vi "Motor with Encoder - Bang Bang.vi"() -> ()   [LabVIEW 2016]
doc: "This example shows how to move a motor connected to an encoder and a wheel, and then read information about the system from an encoder.\n\nThis is an example of how to use feedback (from the encoder) to create an open loop system. If some control method was used, for example using PID, a closed loop system could be created.\n\nThis example expects a USB cable connected from your development PC to the Type B USB Jack (next to the power input) on the roboRIO.\n\nThis example requires the Driver Station to be running with Teleoperated Enabled."
uses:
  <vilib>/Rock Robotics/SystemInterfaces/DIO/FPGA_DIOChannel.ctl
  <vilib>/Rock Robotics/WPI/Encoder/WPI_EncoderType.ctl
  <vilib>/Rock Robotics/SystemInterfaces/DIO/FPGA_DIOPWMChannel.ctl
  <vilib>/Rock Robotics/WPI/Counter/WPI_CounterDigitalInputToDigitalSource.vi
  <vilib>/Rock Robotics/WPI/MotorControl/WPI_MotorControlOpen SPARK.vi
  <vilib>/gmath/NI_Gmath.lvlib
panel:
  in  "Encoder Before Gearbox":bool
  in  "Update RPM":bool
  in  "Error Multiplication Value":dbl
  in  "Lower Limit":dbl=-50.0 format="%#_13g"
  in  "Upper Limit":dbl=50.0 format="%#_13g"
  out "Error":dbl(graph)=-19.827905182603445
  out "Error":dbl=-19.827905182603445
  out "DS Original":dbl=0.6428571428571428
  in  "Neg Drive Signal":dbl=0.6
  in  "Pos Drive Signal":dbl=1.0
  in  "Target RPM":dbl=3300.0
  in  "MS to Wait":u32=10
  out "Loop Time (s)":dbl=0.010378 format="%_6f"
  out "RPM":dbl=3319.8279051826034
  out "XY Graph":cluster{dbl[], dbl[]}[](graph)
  out "Waveform Chart":dbl(graph)=3319.8279051826034
  in  "Motor PWM Channel":T1=enum."PWM 9"
  in  "Number Samples to Average":u8=1 min=1 max=128
  in  "Invert Direction":bool=TRUE
  in  "Decoding Type":T2=enum."2x"
  in  "DistancePerCount (deg)":dbl=0.351563
  in  "Encoder B Channel":T3=enum."DIO 1"
  in  "Encoder A Channel":T3
  in  "Minimum Rate":dbl=20.0
  in  "Stop":bool
  out "Encoder Alarm Status":string="Encoder Moving"
  out "Encoder Direction":string="Forward"
  # "These can be set while running."
  # "Output information."
  # "Set these inputs before running."
  # "This example requires the Driver Station to be running with Teleoperated Enabled."
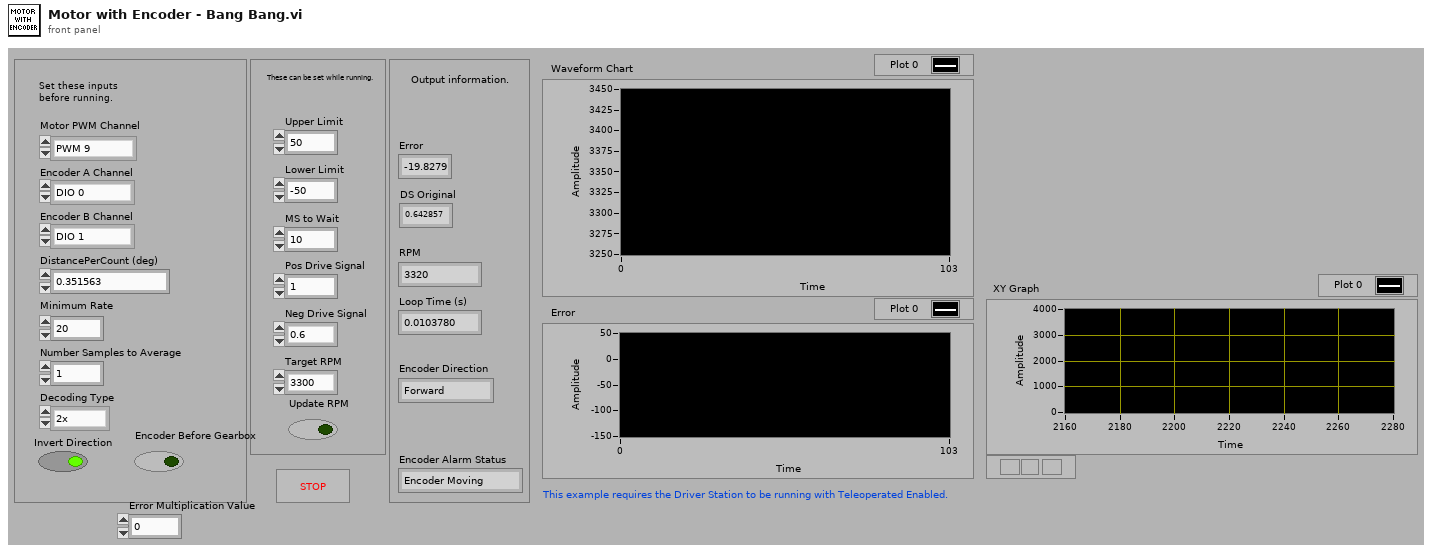
[diagram p1: front panel]
types:
  T1 = typedef "FPGA_DIOPWMChannel.ctl" = enum8{"PWM 0", "PWM 1", "PWM 2", "PWM 3", "PWM 4", "PWM 5", "PWM 6", "PWM 7", "PWM 8", "PWM 9", "PWM MXP 0", "PWM MXP 1", "PWM MXP 2", "PWM MXP 3", "PWM MXP 4", "PWM MXP 5", "PWM MXP 6", "PWM MXP 7", "PWM MXP 8", "PWM MXP 9", "Invalid"}
  T2 = typedef "WPI_EncoderType.ctl" = enum16{"1x", "2x", "4x"}
  T3 = typedef "FPGA_DIOChannel.ctl" = enum8{"DIO 0", "DIO 1", "DIO 2", "DIO 3", "DIO 4", "DIO 5", "DIO 6", "DIO 7", "DIO 8", "DIO 9", "DIO MXP 0", "DIO MXP 1", "DIO MXP 2", "DIO MXP 3", "DIO MXP 4", "DIO MXP 5", "DIO MXP 6", "DIO MXP 7", "DIO MXP 8", "DIO MXP 9", "DIO MXP 10", "DIO MXP 11", "DIO MXP 12", "DIO MXP 13", "DIO MXP 14", "DIO MXP 15", "SPI Port CS1", "SPI Port CS2", "SPI Port CS3", "SPI Port MISO", "SPI Port MOSI", "Invalid"}
  T4 = typedef "WPI_MotorControlDeviceRef.ctl" = cluster{"DeviceStatus":errorcluster, "Type":T5, "PWM":cluster{"PWM Channel":T1, "DeadBand":T6}, "CAN":cluster{"Device Number":u8, "SetOutput VI Ref":variant, "GetOutput VI Ref":variant, "Enable VI Ref":variant, "Disable VI Ref":variant, "Data":variant}, "Invert":bool}
  T5 = typedef "WPI_MotorControlType.ctl" = enum16{"PWM", "CAN"}
  T6 = typedef "WPI_PWMDeadband.ctl" = cluster{"Name":string, "maxPositivePwm":i32, "minPositivePwm":i32, "centerPwm":i32, "maxNegativePwm":i32, "minNegativePwm":i32, "angularRange":u16}
  T7 = typedef "WPI_DigitalInputDevRef.ctl" = cluster{"DevStatus":errorcluster, "DIO Channel":T3}
  T8 = typedef "FPGA_CounterEncoderSourceConvertionLVSourceType.ctl" = cluster{"DevStatus":errorcluster, "AnalogTriggerMode?":bool, "DigitalMode":cluster{"DIO Channel":T9}, "AnalogTriggerMode":cluster{"AnalogTriggerIndex":T10, "OutputType":T11}}
  T9 = typedef "FPGA_DIODigitalSourceChannel.ctl" = enum8{"DIO 0", "DIO 1", "DIO 2", "DIO 3", "DIO 4", "DIO 5", "DIO 6", "DIO 7", "DIO 8", "DIO 9", "DIO MXP 0", "DIO MXP 1", "DIO MXP 2", "DIO MXP 3", "DIO MXP 4", "DIO MXP 5", "DIO MXP 6", "DIO MXP 7", "DIO MXP 8", "DIO MXP 9", "DIO MXP 10", "DIO MXP 11", "DIO MXP 12", "DIO MXP 13", "DIO MXP 14", "DIO MXP 15", "Disabled"}
  T10 = typedef "FPGA_AnalogTriggerIndex.ctl" = enum8{"Trig 0", "Trig 1", "Trig 2", "Trig 3", "Trig 4", "Trig 5", "Trig 6", "Trig 7", "Invalid"}
  T11 = typedef "FPGA_AnalogTriggerOutType.ctl" = enum16{"InWindow", "TriggerState", "Rising", "Falling"}
  T12 = typedef "WPI_EncoderDevRef.ctl" = cluster{"DevStatus":errorcluster, "EncoderIndex":T13, "CounterIndex":T14, "DistancePerCount":dbl, "Decoding Type":T2}
  T13 = typedef "FPGA_EncoderIdx.ctl" = enum8{"Enc 0", "Enc 1", "Enc 2", "Enc 3", "Enc 4", "Enc 5", "Enc 6", "Enc 7", "Invalid"}
  T14 = typedef "FPGA_CounterCtrSystemIndex.ctl" = enum8{"Ctr 0", "Ctr 1", "Ctr 2", "Ctr 3", "Ctr 4", "Ctr 5", "Ctr 6", "Ctr 7", "Invalid"}
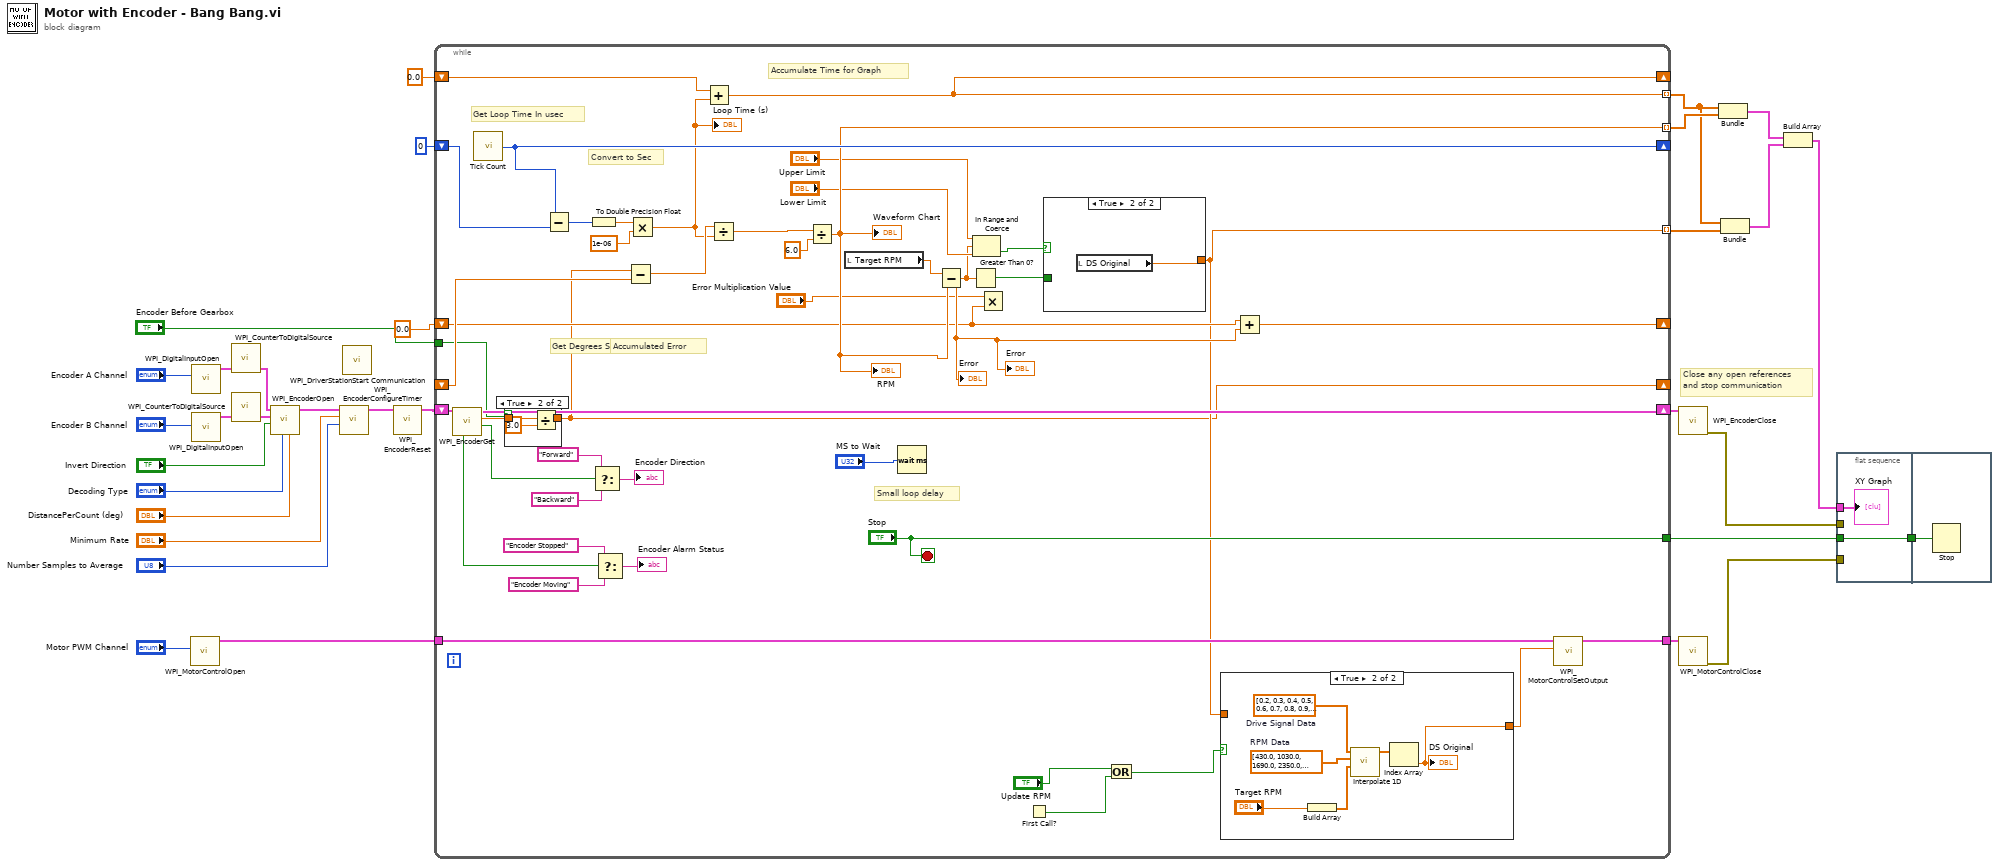
[diagram p0: block diagram]
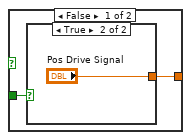
[diagram p4: hidden frame]
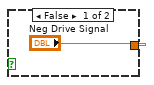
[diagram p5: hidden frame]
diagram:
  # "Close any open references\nand stop communication"
  n1 = call-poly <vilib>:"WPI_MotorControlOpen.vi"("PWM Channel"="Motor PWM Channel") -> ("MotorControlDeviceRef"=w3:T4)  [unwired: 3 in, 7 out]
  n2 = call <vilib>:"WPI_DigitalInputOpen.vi"("DIO Channel"="Encoder A Channel") -> ("DigitalInputDevRef"=w29:T7)  [unwired: 1 in, 9 out]
  n3 = call <vilib>:"WPI_DigitalInputOpen.vi"("DIO Channel"="Encoder B Channel") -> ("DigitalInputDevRef"=w30:T7)  [unwired: 1 in, 9 out]
  n4 = call-poly <vilib>:"WPI_CounterToDigitalSource.vi"("DigitalInputDevRef"=w29) -> ("Digital Source"=w28:T8)  [unwired: 6 out]
  n5 = call-poly <vilib>:"WPI_CounterToDigitalSource.vi"("DigitalInputDevRef"=w30) -> ("Digital Source"=w31:T8)  [unwired: 6 out]
  n6 = call <vilib>:"WPI_EncoderOpen.vi"("DistancePerCount"="DistancePerCount (deg)", "Decoding Type"="Decoding Type", "Invert Direction (False)"="Invert Direction", "BSource"=w31, "ASource"=w28) -> ("EncoderDevRef"=w22:T12)  [unwired: 3 in, 3 out]
  n7 = call <vilib>:"WPI_EncoderConfigureTimer.vi"("Number Samples to Average"="Number Samples to Average", "Minimum Rate"="Minimum Rate", "EncoderDevRef"=w22) -> ("EncoderDevRef"=w15:T12)  [unwired: 1 in, 7 out]
  n8 = call <vilib>:"WPI_DriverStationStart Communication.vi"() -> ()  [unwired: 2 in, 10 out]
  n9 = call <vilib>:"WPI_EncoderReset.vi"("EncoderDevRef"=w15) -> ("EncoderDevRef"=w14:T12)  [unwired: 1 in, 9 out]
  n10 = while {
    shift-right: [w62] -> w32
    shift-left: w14 -> [w65]
    tunnel: ["Stop"] -> w17
    tunnel: w3 -> [w68]
    tunnel: [w67] -> w19
    tunnel: [w49] -> w16 mode=indexing
    tunnel: [w51] -> w10 mode=indexing
    shift-right: [w61] -> _
    shift-left: u32 0 ("Tick Count(uSec)") -> [w60]
    shift-right: [w34] -> _
    shift-left: _ -> [w59]
    shift-right: [w51] -> _
    shift-left: 0.0 ("Tick Count(uSec)") -> [w52]
    tunnel: [w40] -> w9 mode=indexing
    shift-right: [w43] -> _
    shift-left: 0.0 -> [w41]
    tunnel: "Encoder Before Gearbox" -> [w33]
    stop <- "Stop" stop-if-true
    # "Accumulated Error"
    # "Accumulate Time for Graph"
    # "Get Degrees Since Last Cycle"
    # "Convert to Sec"
    # "Get Loop Time In usec"
    # "Small loop delay"
    n11 = call <vilib>:"WPI_EncoderGet.vi"("EncoderDevRef"=w65) -> ("Direction"=w74:bool, "Distance"=w35:dbl, "EncoderDevRef"=w62:T12, "Stopped"=w73:bool)  [unwired: 1 in, 6 out]
    n12 = call "Tick Count"() -> ("Tick Count(uSec)"=w61:u32)
    n13 = case shown="True" w33 {
      tunnel: w35 -> [w77 w80]
      tunnel: [w77 w79] -> w34
      frame False {
      }
      frame True {
        n14 = Divide(x=w80, y=3.0) -> (x/y=w79:dbl)
      }
    }
    n15 = Subtract(x=w61, y=w60) -> (x-y=w58:u32)
    n16 = To Double Precision Float(number=w58) -> (double precision float=w56:dbl)
    n17 = Select(t="Forward", s=w74, f="Backward") -> (s? t:f=→"Encoder Direction":string)
    n18 = Select(t="Encoder Stopped", s=w73, f="Encoder Moving") -> (s? t:f=→"Encoder Alarm Status":string)
    n19 = Subtract(x=w34, y=w59) -> (x-y=w55:dbl)
    n20 = Multiply(x=w56, y=1e-06) -> (x*y=w53:dbl)
    "Loop Time (s)" <- w53
    n21 = Add(x=w52, y=w53) -> (x+y=w51:dbl)
    n22 = Divide(x=w55, y=w53) -> (x/y=w54:dbl)
    n23 = Divide(x=w54, y=6.0) -> (x/y=w49:dbl)
    "Waveform Chart" <- w49
    "RPM" <- w49
    n24 = local read "Target RPM"() -> (w50:dbl)
    n25 = Wait (ms)(milliseconds to wait="MS to Wait") -> ()  [unwired: 1 out]
    n26 = Subtract(x=w50, y=w49) -> (x-y=w44:dbl)
    "Error" <- w44
    "Error" <- w44
    n27 = Greater Than 0?(x=w44) -> (x > 0?=w48:bool)
    n28 = In Range and Coerce(upper limit="Upper Limit", x=w44, lower limit="Lower Limit") -> (In Range?=w45:bool)  [unwired: 1 out]
    n29 = Multiply(x="Error Multiplication Value", y=w41) -> ()  [unwired: 1 out]
    n30 = First Call?() -> (First Call?: T/F=w36:bool)
    n31 = case shown="True" w45 {
      tunnel: w48 -> [w89 _]
      tunnel: [w88 w92] -> w40
      frame False {
        n32 = case shown="True" w89 {
          tunnel: ["Neg Drive Signal" "Pos Drive Signal"] -> w88
          frame False {
          }
          frame True {
          }
        }
      }
      frame True {
        n33 = local read "DS Original"() -> (w92:dbl)
      }
    }
    n34 = Or(x="Update RPM", y=w36) -> (x .or. y?=w37:bool)
    n35 = case shown="True" w37 {
      tunnel: [w81 w82] -> w39
      tunnel: w40 -> [w81 _]
      frame False {
      }
      frame True {
        w87 = dbl[] [430.0, 1030.0, 1690.0, 2350.0, 3000.0, 3700.0, 4400.0, 5000.0, 5550.0]  # RPM Data
        w86 = dbl[] [0.2, 0.3, 0.4, 0.5, 0.6, 0.7, 0.8, 0.9, 1.0]  # Drive Signal Data
        n36 = Build Array("Target RPM") -> (w84:dbl[])
        n37 = call <vilib>:"Interpolate 1D.vi"("xi"=w84, "X"=w87, "Y"=w86) -> ("yi"=w83:dbl[])  [unwired: 6 in, 2 out]
        n38 = Index Array(array=w83) -> (element=w82:dbl)  [unwired: 1 in]
        "DS Original" <- w82
      }
    }
    n39 = Add(x=w41, y=w44) -> (x+y=w43:dbl)
    n40 = call <vilib>:"WPI_MotorControlSetOutput.vi"("Output"=w39, "MotorControlDevRef"=w68) -> ("MotorControlDevRef"=w67:T4)  [unwired: 2 in, 7 out]
  }
  n41 = call <vilib>:"WPI_EncoderClose.vi"("EncoderDevRef"=w32) -> ("error out"=w5:errorcluster)  [unwired: 2 in, 8 out]
  n42 = call <vilib>:"WPI_MotorControlClose.vi"("MotorControlDevRef"=w19) -> ("error out"=w4:errorcluster)  [unwired: 1 in, 9 out]
  n43 = Bundle(w10, w16) -> (w8:cluster{dbl[], dbl[]})  [unwired: 1 in]
  n44 = Bundle(w10, w9) -> (w7:cluster{dbl[], dbl[]})  [unwired: 1 in]
  n45 = Build Array(w8, w7) -> (w6:cluster{dbl[], dbl[]}[])
  n46 = flat-sequence {
    tunnel: w17 -> [w94]
    tunnel: [w94] -> w13
    tunnel: w6 -> [w93]
    tunnel: w5 -> [_]
    tunnel: w4 -> [_]
    tunnel: w13 -> [w95]
    frame #0 {
      "XY Graph" <- w93
    }
    frame #1 {
      n47 = Stop(stop? (T)=w95) -> ()
    }
  }
